vi "Laurel Send Receive.vi"(0 "TCP Network Connection in":refnum<k5>, 2 "Serial VISA (Input)":refnum<visa-resource-name>, 5 "Laurel Serial Commands":T3, 7 "Display Type":T1, 9 "Individual Byte Count":i32=9, 11 "error in (no error)":errorcluster, 12 "All Items Byte Count (Flow Rate)":i32=17, 13 "Connection Type":T2) -> (1 "Single Item":dbl, 3 "Output String":string="0000.00 0004.71", 4 "TCP Network Connection out":refnum<k5>, 6 "Flow Rate (Item 1)":dbl, 8 "Serial VISA (Output)":refnum<visa-resource-name>, 10 "Gallons (Item 2)":dbl, 14 "return count":i32, 15 "error out":errorcluster)   [LabVIEW 2020]
uses:
  Type Definitions/Laurel Serial Commands.ctl
  Type Definitions/Laurel Connection Type.ctl
  Type Definitions/Laurel Display Type.ctl
  <vilib>/Utility/error.llb/whitespace.ctl
panel:
  out "Loop Counter":i32
  out "Send Command out":string
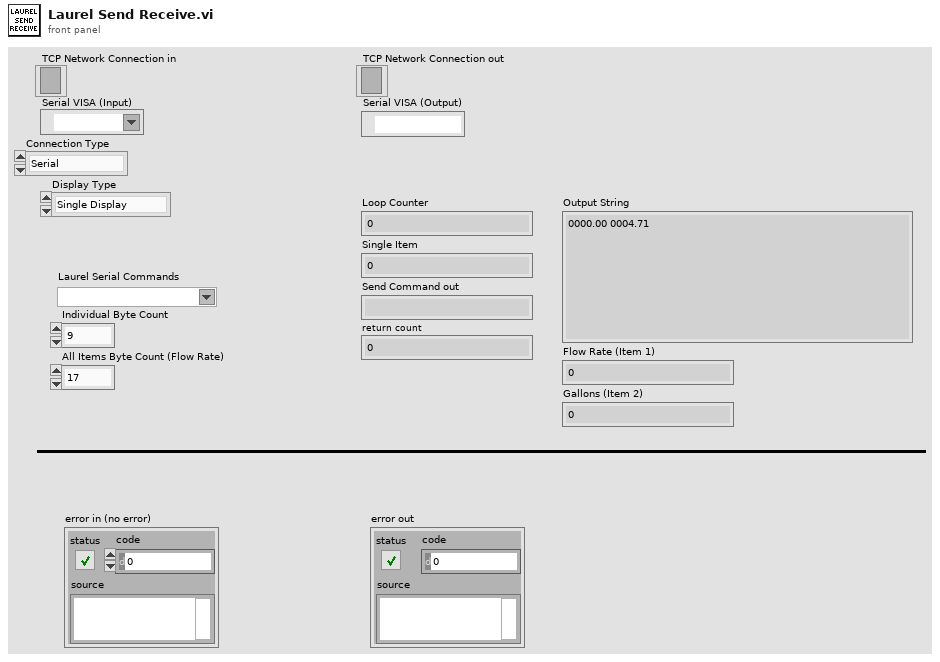
[diagram p1: front panel]
types:
  T1 = typedef "Laurel Display Type.ctl" = enum16{"Single Display", "Dual Display"}
  T2 = typedef "Laurel Connection Type.ctl" = enum16{"Serial", "TCP"}
  T3 = typedef "Laurel Serial Commands.ctl" = string
  T4 = typedef "whitespace.ctl" = u16
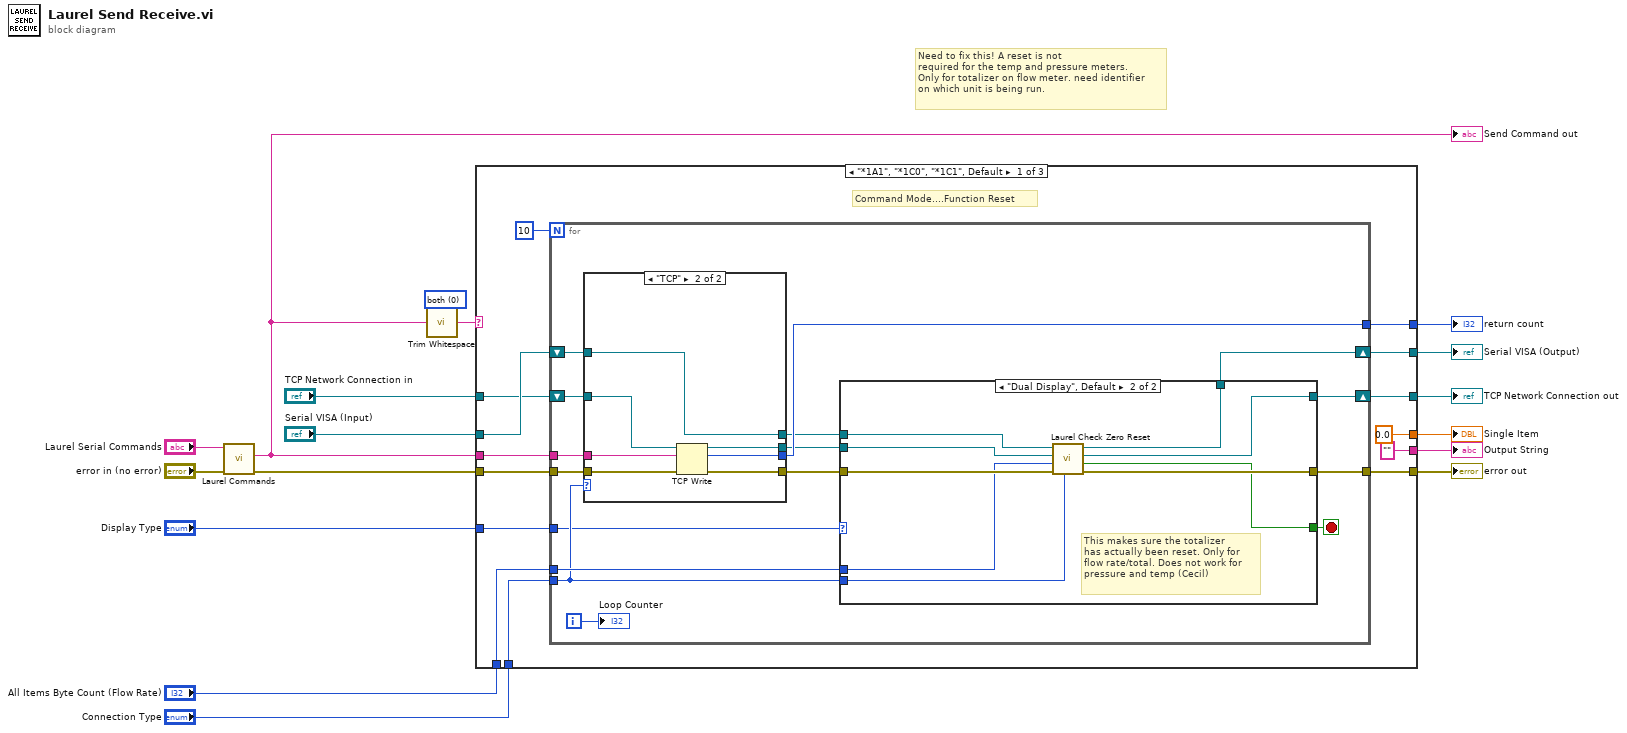
[diagram p0: block diagram]
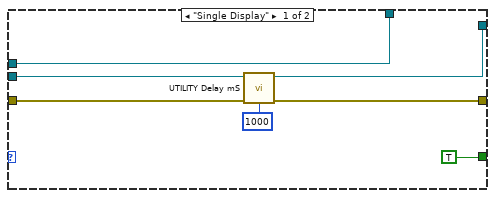
[diagram p2: hidden frame]
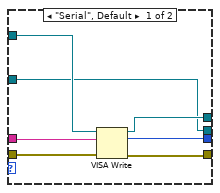
[diagram p3: hidden frame]
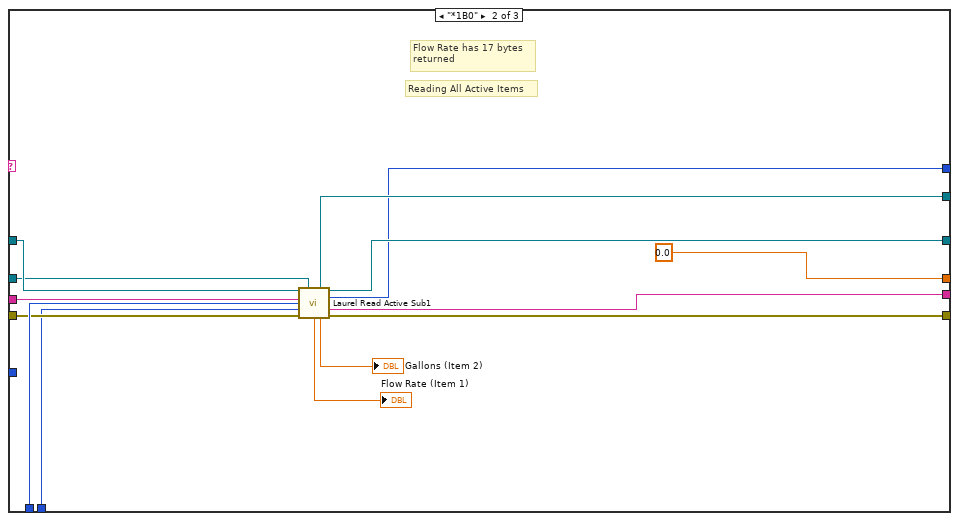
[diagram p4: hidden frame]
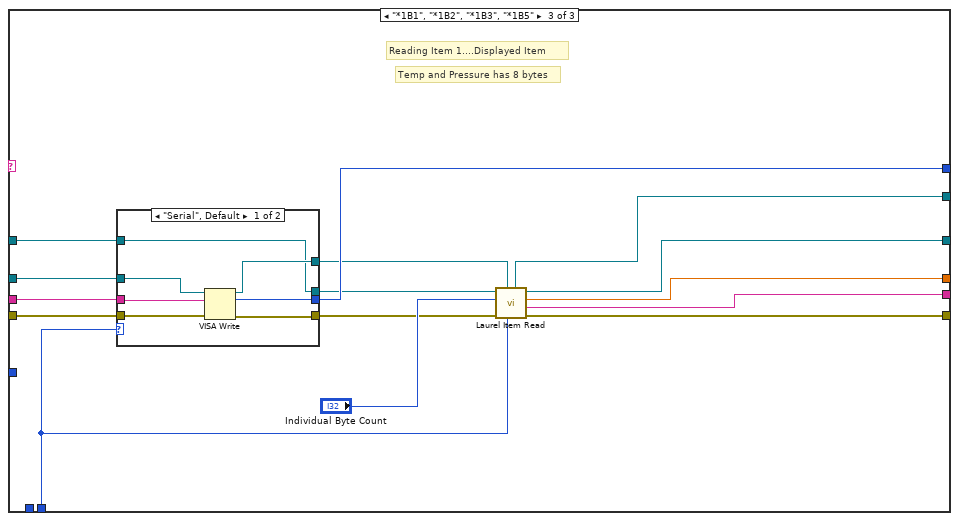
[diagram p5: hidden frame]
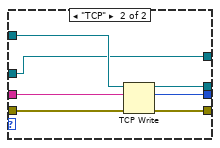
[diagram p6: hidden frame]
diagram:
  w9 = T4 0 items=["both", "start of string", "end of string"] ("location (both)")
  # "Need to fix this! A reset is not \nrequired for the temp and pressure meters. \nOnly for totalizer on flow meter. need identifier\non which unit is being run."
  n1 = call "Laurel Commands.vi"("Error In"="error in (no error)", "Laurel Serial Commands"="Laurel Serial Commands") -> ("Error Out"=w7:errorcluster, "Send Command out"=w6:string)  [unwired: 8 in]
  "Send Command out" <- w6
  n2 = call <vilib>:"Trim Whitespace.vi"("string"=w6, "location (both)"=w9) -> ("trimmed string"=w10:string)
  n3 = case shown="\"*1A1\", \"*1C0\", \"*1C1\", Default" w10 {
    tunnel: [w24 w90 w102] -> w15
    tunnel: [0.0 0.0 w105] -> w17
    tunnel: ["" ("read buffer") w88 w104] -> w14
    tunnel: [w20 w89 w101] -> w16
    tunnel: "Connection Type" -> [w21 w80 w99]
    tunnel: [w23 w86 w100] -> w11
    tunnel: "All Items Byte Count (Flow Rate)" -> [w22 w85 _]
    tunnel: w7 -> [w29 w84 w98]
    tunnel: w6 -> [w28 w81 w97]
    tunnel: "Serial VISA (Input)" -> [w27 w82 w96]
    tunnel: "TCP Network Connection in" -> [w26 w83 w95]
    tunnel: [w25 w79 w94] -> w3
    tunnel: "Display Type" -> [w18 _ _]
    frame "*1A1", "*1C0", "*1C1", Default {
      # "Command Mode....Function Reset"
      n4 = for {
        N: 10 -> [_]
        tunnel: w28 -> [w46]
        tunnel: [w43] -> w25
        tunnel: w22 -> [w38]
        tunnel: w21 -> [w37]
        shift-right: [w40] -> w23
        shift-left: w27 -> [w45]
        shift-right: [w36] -> w20
        shift-left: w26 -> [w44]
        tunnel: w29 -> [w47]
        tunnel: [w35] -> w24
        tunnel: w18 -> [w32]
        i -> [w33]
        stop <- w34 stop-if-true
        n5 = case shown="\"TCP\"" w37 {
          tunnel: [w65 w76] -> w43
          tunnel: [w68 w75] -> w39
          tunnel: w47 -> [w69 w74]
          tunnel: [w63 w73] -> w42
          tunnel: w46 -> [w67 w72]
          tunnel: [w66 w70] -> w41
          tunnel: w45 -> [w64 w70]
          tunnel: w44 -> [w63 w71]
          frame "Serial", Default {
            n6 = VISA Write(VISA resource name=w64, write buffer=w67, error in (no error)=w69) -> (VISA resource name out=w66:refnum<visa-resource-name>, return count=w65:u32, error out=w68:errorcluster)
          }
          frame "TCP" {
            n7 = TCP Write(connection ID=w71, data in=w72, error in (no error)=w74) -> (connection ID out=w73:refnum<k5>, bytes written=w76:i32, error out=w75:errorcluster)  [unwired: 1 in]
          }
        }
        n8 = case shown="\"Dual Display\", Default" w32 {
          tunnel: w42 -> [w48 w62]
          tunnel: w41 -> [w49 w61]
          tunnel: [w49 w60] -> w40
          tunnel: w39 -> [w52 w59]
          tunnel: w38 -> [_ w58]
          tunnel: w37 -> [_ w54]
          tunnel: [w48 w57] -> w36
          tunnel: [w51 w56] -> w35
          tunnel: [TRUE w55] -> w34
          frame "Single Display" {
            n9 = call "UTILITY Delay mS.vi"("Error In"=w52, "milliseconds to wait"=u32 1000) -> ("Error Out"=w51:errorcluster)  [unwired: 13 in]
          }
          frame "Dual Display", Default {
            # "This makes sure the totalizer\nhas actually been reset. Only for\nflow rate/total. Does not work for\npressure and temp (Cecil)"
            n10 = call "Laurel Check Zero Reset.vi"("Connection Type"=w54, "error in (no error)"=w59, "All Items Byte Count (Flow Rate)"=w58, "TCP Network Connection in"=w62, "VISA Refnum in"=w61) -> ("error out"=w56:errorcluster, "Stop Loop?"=w55:bool, "TCP Network Connection out"=w57:refnum<k5>, "VISA Refnum out"=w60:refnum<visa-resource-name>)  [unwired: 3 in]
          }
        }
        "Loop Counter" <- w33
      }
    }
    frame "*1B0" {
      # "Reading All Active Items"
      # "Flow Rate has 17 bytes \nreturned"
      n11 = call "Laurel Read Active Sub1.vi"("TCP Network Connection in"=w83, "Serial VISA"=w82, "Send Command in"=w81, "All Items Byte Count (Flow Rate)"=w85, "Connection Type"=w80, "error in (no error)"=w84) -> ("VISA resource name 2"=w86:refnum<visa-resource-name>, "TCP Network Connection out"=w89:refnum<k5>, "return count"=w79:u32, "trimmed string"=w88:string, "Flow Rate (Item 1)"=→"Flow Rate (Item 1)":dbl, "Gallons (Item 2)"=→"Gallons (Item 2)":dbl, "error out"=w90:errorcluster)  [unwired: 3 in]
    }
    frame "*1B1", "*1B2", "*1B3", "*1B5" {
      # "Reading Item 1....Displayed Item"
      # "Temp and Pressure has 8 bytes"
      n12 = case shown="\"Serial\", Default" w99 {
        tunnel: [w108 w119] -> w94
        tunnel: [w111 w118] -> w91
        tunnel: w98 -> [w112 w117]
        tunnel: [w106 w116] -> w92
        tunnel: w97 -> [w110 w115]
        tunnel: [w109 w113] -> w93
        tunnel: w96 -> [w107 w113]
        tunnel: w95 -> [w106 w114]
        frame "Serial", Default {
          n13 = VISA Write(VISA resource name=w107, write buffer=w110, error in (no error)=w112) -> (VISA resource name out=w109:refnum<visa-resource-name>, return count=w108:u32, error out=w111:errorcluster)
        }
        frame "TCP" {
          n14 = TCP Write(connection ID=w114, data in=w115, error in (no error)=w117) -> (connection ID out=w116:refnum<k5>, bytes written=w119:i32, error out=w118:errorcluster)  [unwired: 1 in]
        }
      }
      n15 = call "Laurel Item Read.vi"("Connection Type"=w99, "VISA resource name"=w93, "error in (no error)"=w91, "byte count"="Individual Byte Count", "TCP Network Connection in"=w92) -> ("error out"=w102:errorcluster, "trimmed string"=w104:string, "Numeric"=w105:dbl, "TCP Network Connection out"=w101:refnum<k5>, "VISA resource name 2"=w100:refnum<visa-resource-name>)  [unwired: 2 in]
    }
  }
  "return count" <- w3
  "Single Item" <- w17
  "TCP Network Connection out" <- w16
  "error out" <- w15
  "Output String" <- w14
  "Serial VISA (Output)" <- w11
